vi "Do Async Auth.vi"(4 "Failed Response (Default)":refnum<class "Response.lvclass">, 5 "Success Response (Default)":refnum<class "Response.lvclass">, 7 "Required Scope(s)":string[](array[string]), 8 "error in (no error)":errorcluster, 9 "Timeout S (60)":dbl=60.0, 10 "Authorization in (New)":refnum<class "Authorization.lvclass">, 11 "OAuth2 in":refnum<class "OAuth2.lvclass">) -> (0 "error out":errorcluster, 1 "Async Authentication":refnum<class "Async Authorization.lvclass">, 3 "OAuth2 out":refnum<class "OAuth2.lvclass">)   [LabVIEW 2020, in "OAuth2.lvlib" / "OAuth2.lvclass"]
doc: "Begins an authorization flow from the beginning. This will open an authorization page in a browser for the user to select an account and approve or deny the authorization. The authorization flow is run asynchronously and this VI returns before the authorization has been completed. To monitor the authorization process an Async Authorization class instance is returned that can provide the state of the authorization flow and be used to retrieve the authorization (or failure) once it completes.\n\nThe authorization defaults to very simple status pages informing the user that they can close the page and return to the application either due to success or failure. HTML content can be customized by providing customized responses.\n\nThe Required Scopes input defines which permissions are needed by the application to perform actions on behalf of the authorizing user. Scopes specified on this VI will be added to any configured with the Request instance that was initialized with the OAuth2 instance.\n\nIf an existing valid but expired authorization is passed in a token refresh will be run that does not require interaction from the user. If the refresh fails, a full authorization flow will be run directing the user to the authorization portal. If using an existing authorization and the user shouldn't be directed to the authorization portal then use <b>Refresh Auth.vi</b> instead."
uses:
  OAuth2.lvclass
  Authorization/Authorization.lvclass
  Async Authorization/Async Authorization.lvclass
  <vilib>/IlluminatedG/IG HTTP Utils/HTTP Utils/Response/Response.lvclass
  OAuth2.lvclass/OAuth2.ctl
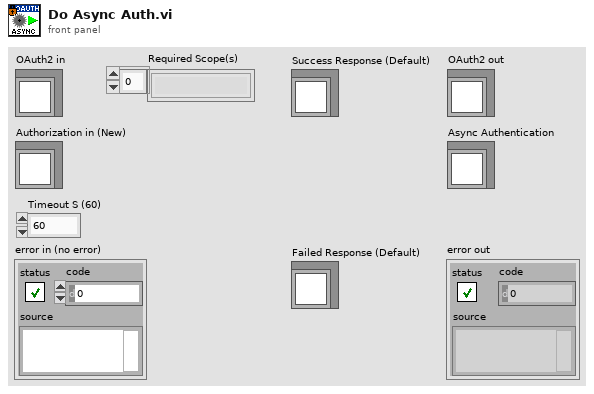
[diagram p1: front panel]
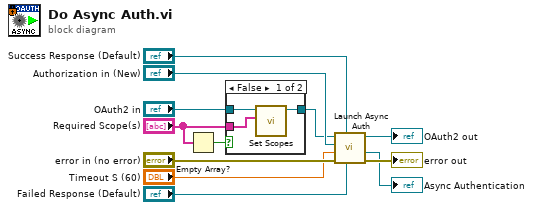
[diagram p0: block diagram]
diagram:
  n1 = Empty Array?(array="Required Scope(s)") -> (empty?=w7:bool)
  n2 = case shown="False" w7 {
    tunnel: "Required Scope(s)" -> [w13 _]
    tunnel: "OAuth2 in" -> [w15 w16]
    tunnel: [w14 w16] -> w3
    frame False {
      n3 = call "Set Scopes.vi"("Scopes"=w13, "OAuth2 in"=w15) -> ("OAuth2 out"=w14:refnum<class "OAuth2.lvclass">)  [unwired: 8 in, 1 out]
    }
    frame True {
    }
  }
  n4 = call "Launch Async Auth.vi"("Failed HTML Response (Default)"="Failed Response (Default)", "Success Response (Default)"="Success Response (Default)", "error in (no error)"="error in (no error)", "Timeout S (60)"="Timeout S (60)", "Authorization in"="Authorization in (New)", "OAuth2 in"=w3) -> ("error out"=→"error out":errorcluster, "Async Authentication"=→"Async Authentication":refnum<class "Async Authorization.lvclass">, "OAuth2 out"=→"OAuth2 out":refnum<class "OAuth2.lvclass">)  [unwired: 3 in]
